vi "View.vi"(8 "error in (no error)":errorcluster, 10 "Debugger":refnum<class "Debug Process.lvclass">, 11 "List View In":refnum<class "Control View.lvclass">) -> (0 "error out":errorcluster, 3 "List View Out":refnum<class "Control View.lvclass">)   [LabVIEW 2020, in "Control View.lvclass"]
uses:
  Control View.lvclass
  C:/Users/anton/Documents/GitHub/triarc-debugger/source/Debug View/Debug View.lvclass
  Process/Debug Process.lvclass
  Debug View/Debug View.lvclass/Debug View.ctl
  Debugger/Debugger.lvclass
  Control View.lvclass/Control View.ctl
  Debug View/Debug View.lvclass
  C:/Users/anton/Documents/GitHub/triarc-debugger/source/Control View/Control View.lvclass
panel:
  in  "Show Selected":bool
  in  "Show Response?":bool=TRUE
  in  "Show Request?":bool=TRUE
  in  "Show Receive?":bool=TRUE
  in  "Show Send?":bool=TRUE
  in  "Refresh?":bool=TRUE
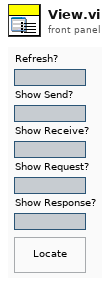
[diagram p1: front panel]
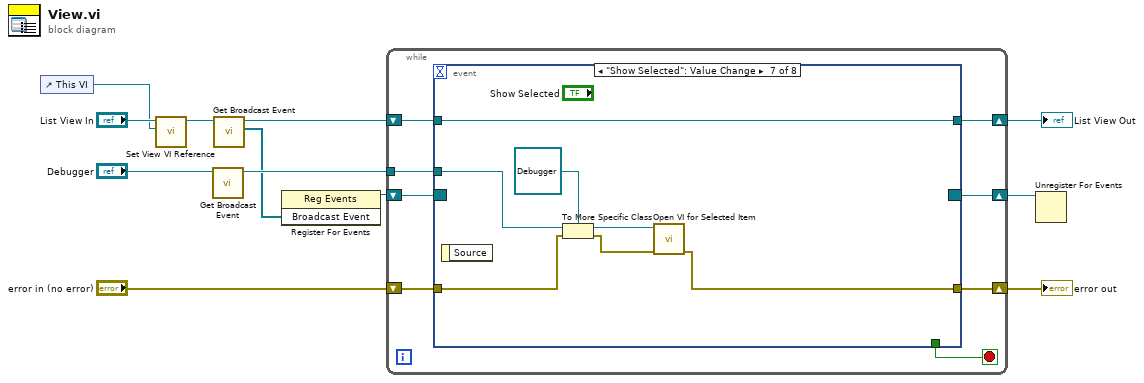
[diagram p0: block diagram]
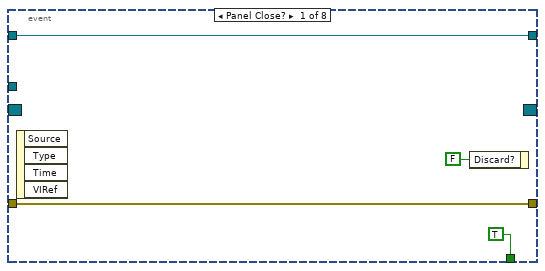
[diagram p2: hidden frame]
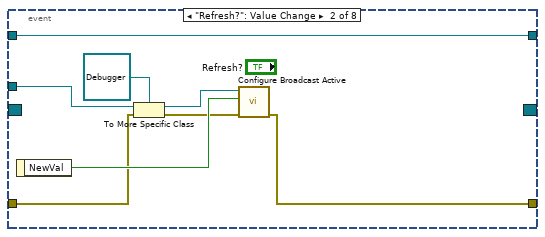
[diagram p3: hidden frame]
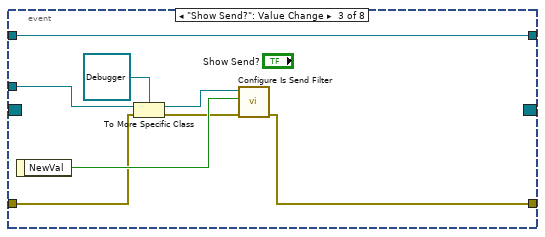
[diagram p4: hidden frame]
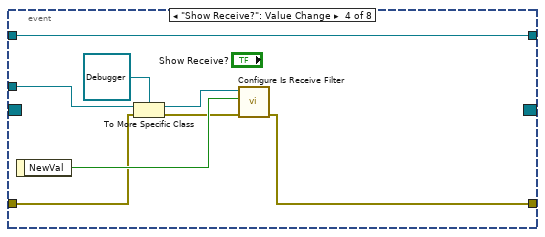
[diagram p5: hidden frame]
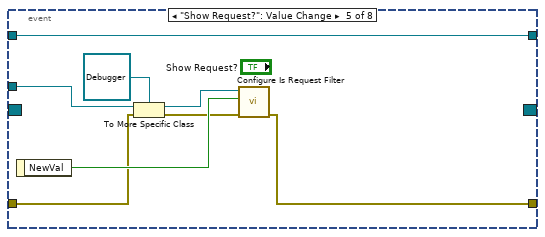
[diagram p6: hidden frame]
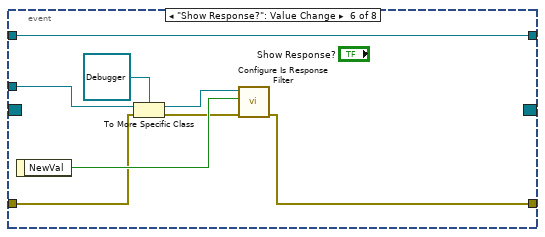
[diagram p7: hidden frame]
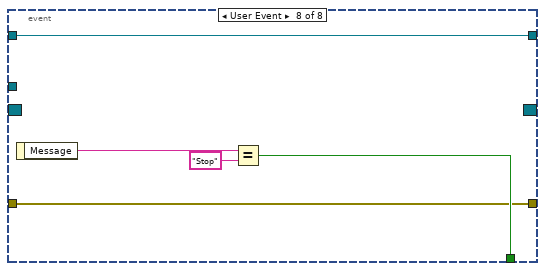
[diagram p8: hidden frame]
diagram:
  n1 = control-ref of="This VI"() -> (w1:refnum<vi>)
  n2 = call "Set View VI Reference.vi"("View VI ref"=w1, "Debug View in"="List View In") -> ("Debug View out"=w2:refnum<class "Control View.lvclass">)  [unwired: 8 in, 1 out]
  n3 = call "Get Broadcast Event.vi"("Process in"="Debugger") -> ("Process out"=w7:refnum<class "Debug Process.lvclass">)  [unwired: 8 in, 2 out]
  n4 = call "Get Broadcast Event.vi"("Debug View In"=w2) -> ("Broadcast Event"=w3:refnum<user-event>[], "Debug View Out"=w4:refnum<class "Control View.lvclass">)  [unwired: 8 in, 1 out]
  n5 = register-events(w3) -> (reference out=w6:refnum<event-registration>)  [unwired: 2 in, 1 out]
  n6 = while {
    shift-right: [w19] -> w12
    shift-left: w4 -> [w20]
    shift-right: [w18] -> w11
    shift-left: "error in (no error)" -> [w17]
    shift-right: [w16] -> w9
    shift-left: w6 -> [w13]
    tunnel: w7 -> [w15]
    stop <- w14 stop-if-true
    n7 = event shown="[6] \"Show Selected\": Value Change" {
      selector: w13 -> [_ _ _ _ _ _ _ _]
      dyn-events: [_ _ _ _ _ _ _ _] -> w16
      timeout: _ -> [_ _ _ _ _ _ _ _]
      tunnel: w20 -> [w24 w25 w33 w41 w49 w57 w71 w72]
      tunnel: [w24 w25 w33 w41 w49 w57 w71 w72] -> w19
      tunnel: [w23 w26 w34 w42 w50 w58 w66 w73] -> w18
      tunnel: w17 -> [w23 w28 w36 w44 w52 w60 w65 w73]
      tunnel: w15 -> [_ w32 w40 w48 w56 w64 w70 _]
      tunnel: [TRUE ("Discard?") _ _ _ _ _ _ w74] -> w14
      event Panel Close? {
        n8 = event-data() -> ()  [unwired: 1 in, 4 out]
        n9 = event-data("Discard?"=FALSE) -> ()  [unwired: 1 in, 1 out]
      }
      event "Refresh?": Value Change {
        n10 = event-data() -> ("NewVal"=w29:bool)  [unwired: 1 in]
        n11 = To More Specific Class(target class=refnum<class "Debugger.lvclass"> refnum ("Debugger Out"), reference=w32, error in=w28) -> (specific class reference=w30:refnum<class "Debugger.lvclass">, error out=w27:errorcluster)
        n12 = call "Configure Broadcast Active.vi"("error in (no error)"=w27, "Active?"=w29, "Debugger In"=w30) -> ("error out"=w26:errorcluster)  [unwired: 7 in, 1 out]
      }
      event "Show Send?": Value Change {
        n13 = event-data() -> ("NewVal"=w37:bool)  [unwired: 1 in]
        n14 = To More Specific Class(target class=refnum<class "Debugger.lvclass"> refnum ("Debugger Out"), reference=w40, error in=w36) -> (specific class reference=w38:refnum<class "Debugger.lvclass">, error out=w35:errorcluster)
        n15 = call "Configure Is Send Filter.vi"("error in (no error)"=w35, "Show Send?"=w37, "Debugger In"=w38) -> ("error out"=w34:errorcluster)  [unwired: 7 in, 1 out]
      }
      event "Show Receive?": Value Change {
        n16 = event-data() -> ("NewVal"=w45:bool)  [unwired: 1 in]
        n17 = To More Specific Class(target class=refnum<class "Debugger.lvclass"> refnum ("Debugger Out"), reference=w48, error in=w44) -> (specific class reference=w46:refnum<class "Debugger.lvclass">, error out=w43:errorcluster)
        n18 = call "Configure Is Receive Filter.vi"("error in (no error)"=w43, "Show Receive?"=w45, "Debugger In"=w46) -> ("error out"=w42:errorcluster)  [unwired: 7 in, 1 out]
      }
      event "Show Request?": Value Change {
        n19 = event-data() -> ("NewVal"=w53:bool)  [unwired: 1 in]
        n20 = To More Specific Class(target class=refnum<class "Debugger.lvclass"> refnum ("Debugger Out"), reference=w56, error in=w52) -> (specific class reference=w54:refnum<class "Debugger.lvclass">, error out=w51:errorcluster)
        n21 = call "Configure Is Request Filter.vi"("error in (no error)"=w51, "Show Request?"=w53, "Debugger In"=w54) -> ("error out"=w50:errorcluster)  [unwired: 7 in, 1 out]
      }
      event "Show Response?": Value Change {
        n22 = event-data() -> ("NewVal"=w61:bool)  [unwired: 1 in]
        n23 = To More Specific Class(target class=refnum<class "Debugger.lvclass"> refnum ("Debugger Out"), reference=w64, error in=w60) -> (specific class reference=w62:refnum<class "Debugger.lvclass">, error out=w59:errorcluster)
        n24 = call "Configure Is Response Filter.vi"("error in (no error)"=w59, "Show Response?"=w61, "Debugger In"=w62) -> ("error out"=w58:errorcluster)  [unwired: 7 in, 1 out]
      }
      event "Show Selected": Value Change {
        n25 = event-data() -> ()  [unwired: 1 in, 1 out]
        n26 = To More Specific Class(target class=refnum<class "Debugger.lvclass"> refnum ("Debugger.lvclass"), reference=w70, error in=w65) -> (specific class reference=w68:refnum<class "Debugger.lvclass">, error out=w67:errorcluster)
        n27 = call "Open VI for Selected Item.vi"("error in (no error)"=w67, "Debugger In"=w68) -> ("error out"=w66:errorcluster)  [unwired: 8 in, 1 out]
      }
      event User Event {
        n28 = event-data() -> ("Message"=w76:string)  [unwired: 1 in]
        n29 = Equal?(x=w76, y="Stop") -> (x = y?=w74:bool)
      }
    }
  }
  "error out" <- w11
  "List View Out" <- w12
  n30 = Unregister For Events(event registration refnum=w9) -> ()  [unwired: 1 in, 1 out]
